vi "Cmd Delete.vi"(8 "error in (no error)":errorcluster, 11 "command reference":T2) -> (0 "error out":errorcluster, 3 "connection reference":T1)   [LabVIEW 2012, in "NI_Database_API_64.lvlib"]
doc: "Frees an object by destroying its associated reference and returns a different reference object. Wire data to the reference input to determine the polymorphic instance to use or manually select the instance."
uses:
  NI_Database_API_64.lvlib
  Cmd ObjectReference.ctl
  Connection.llb/Conn ObjectReference.ctl
  <vilib>/Utility/_goopsup.llb/GOOP Object Repository Method.ctl
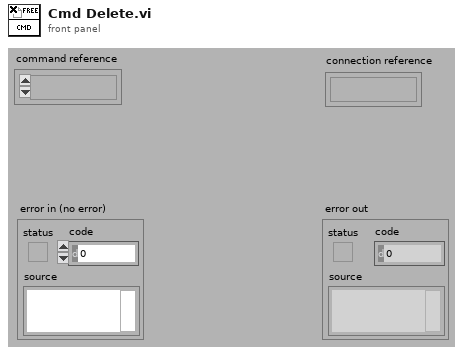
[diagram p1: front panel]
types:
  T1 = typedef "NI_Database_API_64.lvlib/Conn ObjectReference.ctl" = refnum<k1>
  T2 = typedef "NI_Database_API_64.lvlib/Cmd ObjectReference.ctl" = refnum<k1>
  T3 = typedef "GOOP Object Repository Method.ctl" = enum16{"Create", "GetCopy", "GetModify", "Set", "Destroy", "Create Static", "Get All Refs", "Reset", "Get Statistics"}
  T4 = typedef "NI_Database_API_64.lvlib/Cmd DataMembers.ctl" = cluster{"ADODB._Command":refnum<k7>, "Connection":T1}
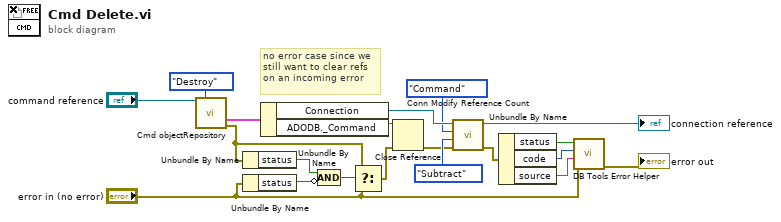
[diagram p0: block diagram]
diagram:
  # "no error case since we\nstill want to clear refs\non an incoming error"
  n1 = call "Cmd objectRepository.vi"("command reference"="command reference", "method"=GOOP_Object_Repository_Method."Destroy") -> ("classDataOut"=w7:T4, "error out"=w8:errorcluster)  [unwired: 5 in, 7 out]
  n2 = Unbundle By Name(w8) -> ("status"=w10:bool)
  n3 = Unbundle By Name("error in (no error)") -> ("status"=w11:bool)
  n4 = Unbundle By Name(w7) -> ("Connection"=w16:T1, "ADODB._Command"=w17:refnum<k7>)
  n5 = Compound Arithmetic op=AND(w10, invert w11) -> (w12:bool)
  n6 = Select(t=w8, s=w12, f="error in (no error)") -> (s? t:f=w6:errorcluster)
  n7 = Close Reference(reference=w17, error in (no error)=w6) -> (error out=w13:errorcluster)
  n8 = call "Conn Modify Reference Count.vi"("error in (no error)"=w13, "operation"=enum16{"Add", "Subtract"}."Subtract" ("Operation"), "object"=enum16{"Recordset", "Command"}."Command" ("Object"), "connection reference"=w16) -> ("error out"=w2:errorcluster, "connection reference out"=→"connection reference":T1)  [unwired: 4 out]
  n9 = Unbundle By Name(w2) -> ("status"=w4:bool, "code"=w3:i32, "source"=w5:string)
  n10 = call "DB Tools Error Helper.vi"("Overriding error or warning"="error in (no error)", "source"=w5, "code"=w3, "status"=w4) -> ("error out"=→"error out":errorcluster)  [unwired: 7 out]
